vi "Get Unvisited Neighbors.vi"(7 "Unvisited":bool[][](array[boolean]), 11 "Current Point":i32[](array[numeric])) -> (3 "Unvisited Neighbors":cluster{"X":i32, "Y":i32}[](array[cluster]))   [LabVIEW 2021]
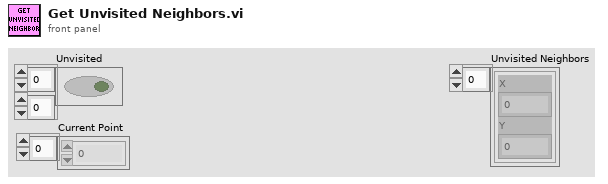
[diagram p1: front panel]
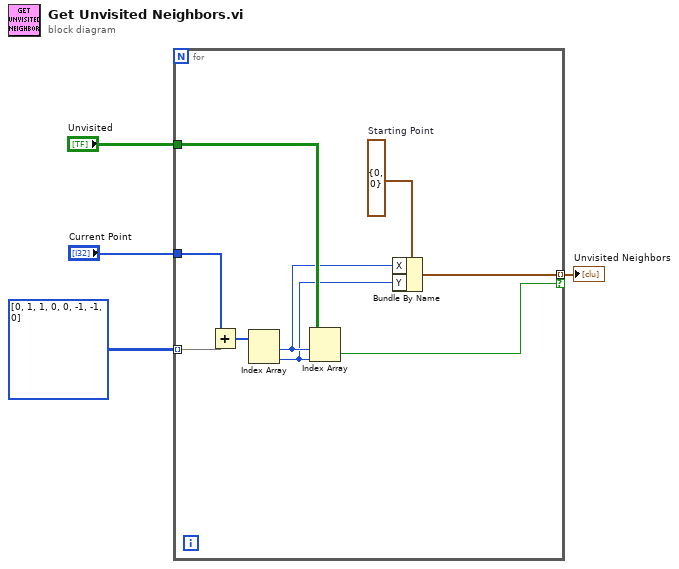
[diagram p0: block diagram]
diagram:
  n1 = for {
    tunnel: "Current Point" -> [w12]
    tunnel: i32[][] [[0, 1], [1, 0], [0, -1], [-1, 0]] -> [w13] mode=indexing
    tunnel: "Unvisited" -> [w10]
    tunnel: [w6] -> w1 mode=indexing if=w5
    w9 = cluster{"X":i32, "Y":i32} {"X"=0, "Y"=0}  # Starting Point
    n2 = Add(x=w12, y=w13) -> (x+y=w11:i32[])
    n3 = Index Array(array=w11) -> (element #1=w8:i32, element #2=w7:i32)  [unwired: 2 in]
    n4 = Index Array(array=w10, index (row)=w8, index (col)=w7) -> (element=w5:bool)
    n5 = Bundle By Name(cluster=w9, "X"=w8, "Y"=w7) -> (w6:cluster{"X":i32, "Y":i32})
  }
  "Unvisited Neighbors" <- w1
